vi "hardware names - global.vi"() -> ()   [LabVIEW 2014]
panel:
  in  "Microscope software version":string
  in  "Microscope":string
  in  "Camera":string
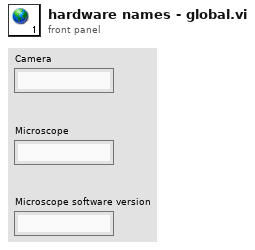
[diagram p1: front panel]
diagram:
